vi "PID Process Value and Setpoint.vi"(4 "Allowable Error Disables Accumulator":bool=TRUE, 6 "PID Config":T1={"Gains"={"P"=1.0, "I"=0.01, "D"=0.0, "F"=0.0}, "Error Allowed"={"High"=0.1, "Low"=-0.1}, "I Zone"={"High"=10.0, "Low"=-10.0}, "Max Out"={"FWD"=100.0, "REV"=-100.0}, "Max I Accu"={"High"=0.0, "Low"=0.0}, "CL Ramp Rate (S)"=0.0} {"Max I Accu"."Low" format="%#.8f"; "Max I Accu"."High" format="%#.8f"; "Gains"."F" format="%#.8f"; "Gains"."D" format="%#.8f"; "Gains"."I" format="%#.8f"; "Gains"."P" format="%#.8f"; "Error Allowed"."Low" format="%#.8f"; "Error Allowed"."High" format="%#.8f"; "I Zone"."Low" format="%#.8f"; "I Zone"."High" format="%#.8f"; "Max Out"."REV" format="%.2f"; "Max Out"."FWD" format="%.2f"}, 7 "Target Cycle Time(S)":dbl=0.05 format="%.3f", 8 "Setpoint":dbl format="%.2f", 11 "Process Variable":dbl format="%.2f") -> (0 "PID Enabled Out":bool, 2 "Error Out":dbl, 3 "Output Out":dbl format="%.2f", 5 "Time Mulitplyer Out":dbl)   [LabVIEW 2023]
uses:
  <vilib>/addons/control/pid/NI_PID_pid.lvlib
  <vilib>/addons/control/pid/pid.llb/PID (DBL).vi
  Shared Code/TypeDefs/Cluster_High-Low.ctl
  Shared Code/TypeDefs/Cluster_PID Gains.ctl
  Shared Code/TypeDefs/Cluster_SRX SLOT PID Config.ctl
  Shared Code/TypeDefs/Cluster_FWD  REV Values.ctl
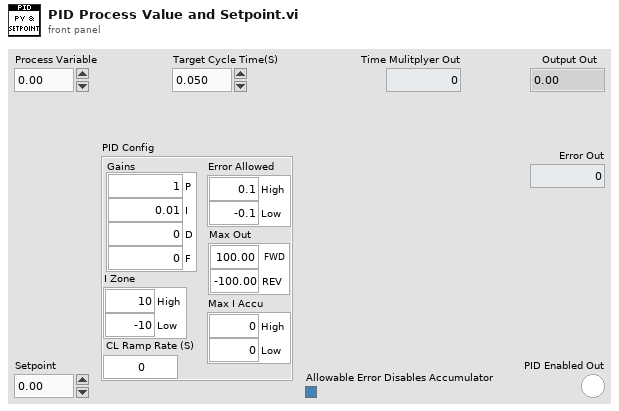
[diagram p1: front panel]
types:
  T1 = typedef "Cluster_PID Config.ctl" = cluster{"Gains":T2, "Error Allowed":T3, "I Zone":T3, "Max Out":T4, "Max I Accu":T3, "CL Ramp Rate (S)":dbl}
  T2 = typedef "Cluster_PID Gains.ctl" = cluster{"P":dbl, "I":dbl, "D":dbl, "F":dbl}
  T3 = typedef "Cluster_High-Low.ctl" = cluster{"High":dbl, "Low":dbl}
  T4 = typedef "Cluster_FWD  REV Values.ctl" = cluster{"FWD":dbl, "REV":dbl}
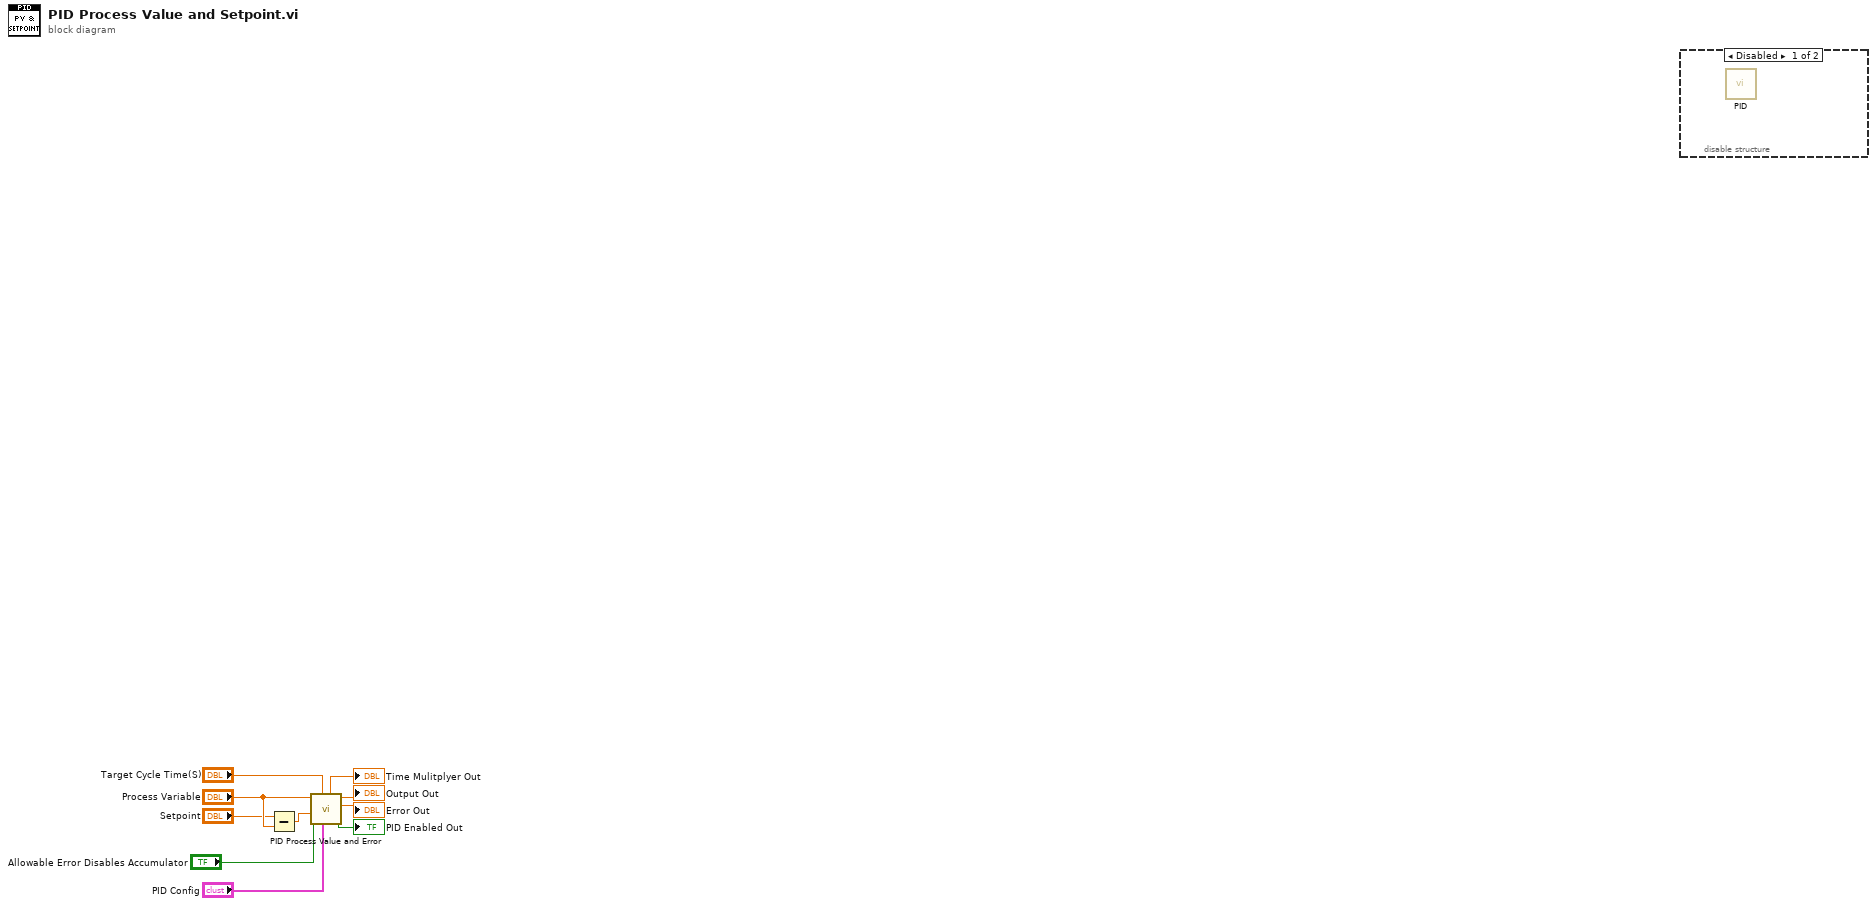
[diagram p0: block diagram]
diagram:
  n1 = Subtract(x="Setpoint", y="Process Variable") -> (x-y=w2:dbl)
  n2 = call "PID Process Value and Error.vi"("PID Config"="PID Config", "Target Cycle Time(S)"="Target Cycle Time(S)", "Allowable Error Disables Accumulator"="Allowable Error Disables Accumulator", "ERROR"=w2, "Process Variable"="Process Variable") -> ("PID Enabled Out"=→"PID Enabled Out":bool, "Error Out"=→"Error Out":dbl, "Output Out"=→"Output Out":dbl, "Time Mulitplyer Out"=→"Time Mulitplyer Out":dbl)  [unwired: 2 in, 1 out]
  n3 = disable-structure shown="Disabled" {
    frame Disabled {
      n4 = call-poly <vilib>:"PID.vi"() -> ()  [unwired: 10 in, 2 out]
    }
    frame Enabled {
    }
  }
